vi "Bertta_v09_97.vi"() -> ()   [LabVIEW 2016]
uses:
  x64/Debug/BERTTA.dll
panel:
  out "element":bool
  out "Started:":string
  in  "SHUTDOWN":bool
  in  "MASTER CONTROL":bool
  in  "Tab Control":T1(tab)
  out "Output File":path caption="selected path"
  in  "Browse folder":path=path "" caption="start path"
  in  "Read Seq":bool
  in  "Save Seq":bool
  in  "Configuration file":path=path "C:/Users/shresplab/Desktop/BerttaConfiguration.lvm" caption="Filename"
  in  "OK Button 2":bool
  out "Boolean":bool
  in  "User (initials)":string
  in  "Project name":string
  in  "Description":string
  out "PUMP1":bool
  out "Target amount":dbl
  out "Scale weight":dbl
  out "Amount now":dbl
  out "Flow rate":dbl
  out "Time to target":dbl format="%<%H:%M:%S>t"
  out "Current step":dbl
  out "Target":dbl
  out "Amount now":dbl
  out "Amount now":dbl
  out "Target":dbl
  out "Current step":dbl
  out "Time to target":dbl format="%<%H:%M:%S>t"
  out "Flow rate":dbl
  out "Amount now":dbl
  out "Scale weight":dbl
  out "Target amount":dbl
  out "PUMP2":bool
  out "Sensor OK 6":bool
  out "Sensor OK 5":bool
  out "Sensor OK 4":bool
  out "Sensor OK 3":bool
  in  "OK Button":bool
  in  "Add comment":string
  out "PUMP3":bool
  out "Target amount":dbl
  out "Scale weight":dbl
  out "Amount now":dbl
  out "Flow rate":dbl
  out "Time to target":dbl format="%<%H:%M:%S>t"
  out "Current step":dbl
  out "Target":dbl
  out "Amount now":dbl
  out "Tr":dbl
  out "Tj in":dbl
  out "Tj out":dbl
  out "T set":dbl
  out "Current step":i32
  out "RPM":dbl
  out "Torque 2":dbl
  out "Waveform Chart 5":dynamicdata(graph)
  out "Waveform Chart 6":dynamicdata(graph)
  out "Waveform Chart 7":dynamicdata(graph)
  in  "Tab Control 2":T2(tab)
  out "Waveform Chart 3":dynamicdata(graph)
  out "Waveform Chart 8":dynamicdata(graph)
  out "Waveform Chart 11":dynamicdata(graph)
  out "Waveform Chart 13":dynamicdata(graph)
  out "Waveform Chart 9":dynamicdata(graph)
  out "Table":string[][](table)=[["14.8.2017 18.06.59", "0,000000", "417,670000", "-0,150000", "1,000000", "22,220000", "23,366837", "23,574959", "23,985852", "23,690000", "240,000000", "4,000000", "0,000000", "397,000000", "-397,000000", "1,000000"], ["14.8.2017 18.07.06", "0,000000", "417,640000", "-0,120000", "1,000000", "22,220000", "23,763115", "23,906257", "23,985694", "23,680000", "240,000000", "4,000000", "0,000000", "397,000000", "-397,000000", "1,000000"], ["14.8.2017 18.07.13", "0,000000", "417,640000", "-0,120000", "1,000000", "22,220000", "23,965922", "24,013440", "23,984906", "23,670000", "240,000000", "4,100000", "3,000000", "397,000000", "-397,000000", "1,000000"], ["14.8.2017 18.07.21", "0,000000", "417,640000", "-0,120000", "1,000000", "22,220000", "23,943860", "23,900110", "23,987113", "23,670000", "240,000000", "4,000000", "0,000000", "397,000000", "-397,000000", "1,000000"], ["14.8.2017 18.07.28", "0,000000", "417,640000", "-0,120000", "1,000000", "22,220000", "23,736328", "23,600018", "23,989004", "23,660000", "240,000000", "4,000000", "0,000000", "397,000000", "-397,000000", "1,000000"], ["14.8.2017 18.07.36", "0,000000", "417,640000", "-0,120000", "1,000000", "22,220000", "23,480910", "23,324538", "23,991053", "23,660000", "240,000000", "4,000000", "0,000000", "397,000000", "-397,000000", "1,000000"], ["14.8.2017 18.07.43", "0,000000", "417,640000", "-0,120000", "2,000000", "22,220000", "23,195579", "23,008270", "23,999093", "23,650000", "240,000000", "4,000000", "0,000000", "397,000000", "-397,000000", "1,000000"], ["14.8.2017 18.07.51", "0,000000", "417,650000", "-417,650000", "1,000000", "22,220000", "22,862541", "22,649021", "24,003979", "23,650000", "240,000000", "4,000000", "0,000000", "397,000000", "-397,000000", "2,000000"], ["14.8.2017 18.07.58", "0,000000", "417,640000", "0,010000", "1,000000", "22,220000", "22,541353", "22,354878", "24,005398", "23,650000", "240,000000", "4,000000", "0,000000", "397,000000", "-397,000000", "1,000000"], ["14.8.2017 18.08.06", "0,000000", "417,640000", "0,010000", "1,000000", "22,220000", "22,347931", "22,253738", "24,007605", "23,640000", "240,000000", "4,100000", "0,000000", "397,000000", "-397,000000", "1,000000"], ["14.8.2017 18.08.13", "0,000000", "417,640000", "0,010000", "1,000000", "22,220000", "22,329030", "22,302102", "24,006028", "23,640000", "240,000000", "4,000000", "0,000000", "395,820000", "-395,820000", "1,000000"], ["14.8.2017 18.08.20", "0,000000", "417,640000", "0,010000", "1,000000", "22,220000", "22,466849", "22,511320", "24,002403", "23,630000", "240,000000", "4,000000", "0,000000", "395,830000", "-0,010000", "1,000000"], ["14.8.2017 18.08.28", "0,000000", "417,640000", "0,010000", "1,000000", "22,220000", "22,707062", "22,835101", "24,000984", "23,620000", "240,000000", "4,000000", "0,000000", "395,830000", "-0,010000", "1,000000"], ["14.8.2017 18.08.35", "0,000000", "417,640000", "0,010000", "1,000000", "22,220000", "23,054104", "23,232979", "24,001299", "23,600000", "240,000000", "4,000000", "0,000000", "395,830000", "-0,010000", "1,000000"], ["14.8.2017 18.08.43", "0,000000", "417,640000", "0,010000", "1,000000", "22,220000", "23,412371", "23,522793", "24,002560", "23,590000", "240,000000", "4,000000", "0,000000", "395,820000", "0,000000", "1,000000"], ["14.8.2017 18.08.51", "0,000000", "417,640000", "0,010000", "1,000000", "22,220000", "23,596247", "23,656125", "24,003821", "23,580000", "240,000000", "4,000000", "0,000000", "395,820000", "0,000000", "1,000000"]]
  out "Boolean 4":bool
  out "Boolean 3":bool
  out "Boolean 2":bool
  in  "Reset 6":bool
  in  "Manual/Ramp":bool=TRUE
  in  "Array":dbl[][](array[numeric])=[[20.0, 0.0], [20.0, 0.0], [20.0, 0.0]]
  in  "?":bool
  in  "Time":dbl format="Time to target (min):                %#_g"
  out "Current temp":dbl format="Current temperature (S1):   %#_6g"
  in  "OK Button 3":bool
  in  "T ext / T ext 2":enum32{"Sensor 1", "Sensor 2"}(radio)
  out "Sensor OK":bool
  in  "T fail":dbl=20.0 format="Failsafe temperature:              %#_g"
  in  "Setpoint":dbl=20.0 format="Temperature target:                %#_6g"
  in  "Manual select":T3(radio)
  out "Waveform Chart":dynamicdata(graph)
  out "T external 2":dbl format="Current temperature (S2):    %#_g"
  in  "UPDATE TEMP":bool
  out "Led11 5":bool
  out "RPM":dbl format="%_4f"
  out "Led10 3":bool
  out "Led9 3":bool
  out "Led8 3":bool
  out "Led7 3":bool
  out "Led6 3":bool
  out "Led5 3":bool
  out "Led4 3":bool
  out "Led3 3":bool
  out "Led2 3":bool
  out "Led1 3":bool
  in  "PumpSeq 4":dbl[][](array[numeric])=[[0.0, 0.0, 0.0, 0.0, 0.0, 0.0, 0.0, 0.0, 0.0, 0.0], [0.0, 0.0, 0.0, 0.0, 0.0, 0.0, 0.0, 0.0, 0.0, 0.0], [0.0, 0.0, 0.0, 0.0, 0.0, 0.0, 0.0, 0.0, 0.0, 0.0], [0.0, 0.0, 0.0, 0.0, 0.0, 0.0, 0.0, 0.0, 0.0, 0.0], [0.0, 0.0, 0.0, 0.0, 0.0, 0.0, 0.0, 0.0, 0.0, 0.0], [0.0, 0.0, 0.0, 0.0, 0.0, 0.0, 0.0, 0.0, 0.0, 0.0], [0.0, 0.0, 0.0, 0.0, 0.0, 0.0, 0.0, 0.0, 0.0, 0.0], [0.0, 0.0, 0.0, 0.0, 0.0, 0.0, 0.0, 0.0, 0.0, 0.0], [0.0, 0.0, 0.0, 0.0, 0.0, 0.0, 0.0, 0.0, 0.0, 0.0], [0.0, 0.0, 0.0, 0.0, 0.0, 0.0, 0.0, 0.0, 0.0, 0.0]]
  in  "?":bool
  out "Flow rate (g/min)":dbl
  out "Scale reading":dbl
  out "Step amount now":dbl
  in  "Grams / min":dbl
  out "Waveform Chart 14":dynamicdata(graph)
  in  "?":bool
  out "Total amount now":dbl
  out "Led11 4":bool
  in  "Reset 5":bool
  out "Elapsed / step":i32
  out "Time to target":dbl format="%<%H:%M:%S>t"
  in  "OK Button 4":bool
  out "Led11":bool
  out "RPM":dbl format="%_4f"
  out "Led10":bool
  out "Led9":bool
  out "Led8":bool
  out "Led7":bool
  out "Led6":bool
  out "Led5":bool
  out "Led4":bool
  out "Led3":bool
  out "Led2":bool
  out "Led1":bool
  in  "PumpSeq 2":dbl[][](array[numeric])=[[0.0, 0.0, 0.0, 0.0, 0.0, 0.0, 0.0, 0.0, 0.0, 0.0], [0.0, 0.0, 0.0, 0.0, 0.0, 0.0, 0.0, 0.0, 0.0, 0.0], [0.0, 0.0, 0.0, 0.0, 0.0, 0.0, 0.0, 0.0, 0.0, 0.0], [0.0, 0.0, 0.0, 0.0, 0.0, 0.0, 0.0, 0.0, 0.0, 0.0], [0.0, 0.0, 0.0, 0.0, 0.0, 0.0, 0.0, 0.0, 0.0, 0.0], [0.0, 0.0, 0.0, 0.0, 0.0, 0.0, 0.0, 0.0, 0.0, 0.0], [0.0, 0.0, 0.0, 0.0, 0.0, 0.0, 0.0, 0.0, 0.0, 0.0], [0.0, 0.0, 0.0, 0.0, 0.0, 0.0, 0.0, 0.0, 0.0, 0.0], [0.0, 0.0, 0.0, 0.0, 0.0, 0.0, 0.0, 0.0, 0.0, 0.0], [0.0, 0.0, 0.0, 0.0, 0.0, 0.0, 0.0, 0.0, 0.0, 0.0]]
  in  "?":bool
  out "Flow rate (g/min)":dbl
  out "Scale reading":dbl
  out "Step amount now":dbl
  in  "Grams / min":dbl
  out "Waveform Chart 10":dynamicdata(graph)
  in  "?":bool
  out "Total amount now":dbl
  out "Led11":bool
  in  "Reset 3":bool
  out "Elapsed / step":i32
  out "Time to target":dbl format="%<%H:%M:%S>t"
  in  "OK Button 5":bool
  out "Led11 3":bool
  out "RPM":dbl format="%_4f"
  out "Led10 2":bool
  out "Led9 2":bool
  out "Led8 2":bool
  out "Led7 2":bool
  out "Led6 2":bool
  out "Led5 2":bool
  out "Led4 2":bool
  out "Led3 2":bool
  out "Led2 2":bool
  out "Led1 2":bool
  in  "PumpSeq 3":dbl[][](array[numeric])=[[0.0, 0.0, 0.0, 0.0, 0.0, 0.0, 0.0, 0.0, 0.0, 0.0], [0.0, 0.0, 0.0, 0.0, 0.0, 0.0, 0.0, 0.0, 0.0, 0.0], [0.0, 0.0, 0.0, 0.0, 0.0, 0.0, 0.0, 0.0, 0.0, 0.0], [0.0, 0.0, 0.0, 0.0, 0.0, 0.0, 0.0, 0.0, 0.0, 0.0], [0.0, 0.0, 0.0, 0.0, 0.0, 0.0, 0.0, 0.0, 0.0, 0.0], [0.0, 0.0, 0.0, 0.0, 0.0, 0.0, 0.0, 0.0, 0.0, 0.0], [0.0, 0.0, 0.0, 0.0, 0.0, 0.0, 0.0, 0.0, 0.0, 0.0], [0.0, 0.0, 0.0, 0.0, 0.0, 0.0, 0.0, 0.0, 0.0, 0.0], [0.0, 0.0, 0.0, 0.0, 0.0, 0.0, 0.0, 0.0, 0.0, 0.0], [0.0, 0.0, 0.0, 0.0, 0.0, 0.0, 0.0, 0.0, 0.0, 0.0]]
  in  "?":bool
  out "Flow rate (g/min)":dbl
  out "Scale reading":dbl
  out "Step amount now":dbl
  in  "Grams / min":dbl
  out "Waveform Chart 12":dynamicdata(graph)
  in  "?":bool
  out "Total amount now":dbl
  out "Led11 2":bool
  in  "Reset 4":bool
  out "Elapsed / step":i32
  out "Time to target":dbl format="%<%H:%M:%S>t"
  in  "OK Button 6":bool
  in  "Remote / Manual":bool
  in  "Set RPM":i32
  out "RPM":dbl
  out "Torque":dbl
  out "Waveform Chart 4":dynamicdata(graph)
  in  "OK Button 7":bool
  out "PortDev out":dbl[](array[numeric])
  in  "Save PortDev":bool
  out "PortDev in":dbl[](array[numeric])
  in  "dev1":i32
  in  "dev2":i32
  in  "dev3":i32
  in  "dev4":i32
  in  "dev5":i32
  in  "dev6":i32
  in  "dev8":i32
  in  "port1":i32
  in  "port2":i32
  in  "port3":i32
  in  "port4":i32
  in  "port5":i32
  in  "port6":i32
  in  "port7":i32
  in  "port8":i32
  in  "dev7":i32
  in  "Treshold (T/C)":dbl=0.5
  out "DAQ 9217 (PT100)":errorcluster
  out "Config File":dbl[][](array[numeric])
  # "Temperature sensor:"
  # "Manual control:"
  # "PUMP & SCALE 1"
  # "STEP"
  # "TOTAL"
  # "PUMP & SCALE 2"
  # "STEP"
  # "TOTAL"
  # "PUMP & SCALE 3"
  # "STEP"
  # "TOTAL"
  # "Temperature control parameter"
  # "Secondary temperature sensor"
  # "Temp target"
  # "Time target"
  # "Grams    /   min"
  # "End of sequence"
  # "Manual control"
  # "Grams    /   min"
  # "End of sequence"
  # "Manual control"
  # "Grams    /   min"
  # "End of sequence"
  # "Manual control"
  # "dev1 and dev2 always to port1 and 2\nport1 = port2 = Lauda\n\ndev3 and dev4 always to port3 and port4\nport3 = port4 = Heidolph"
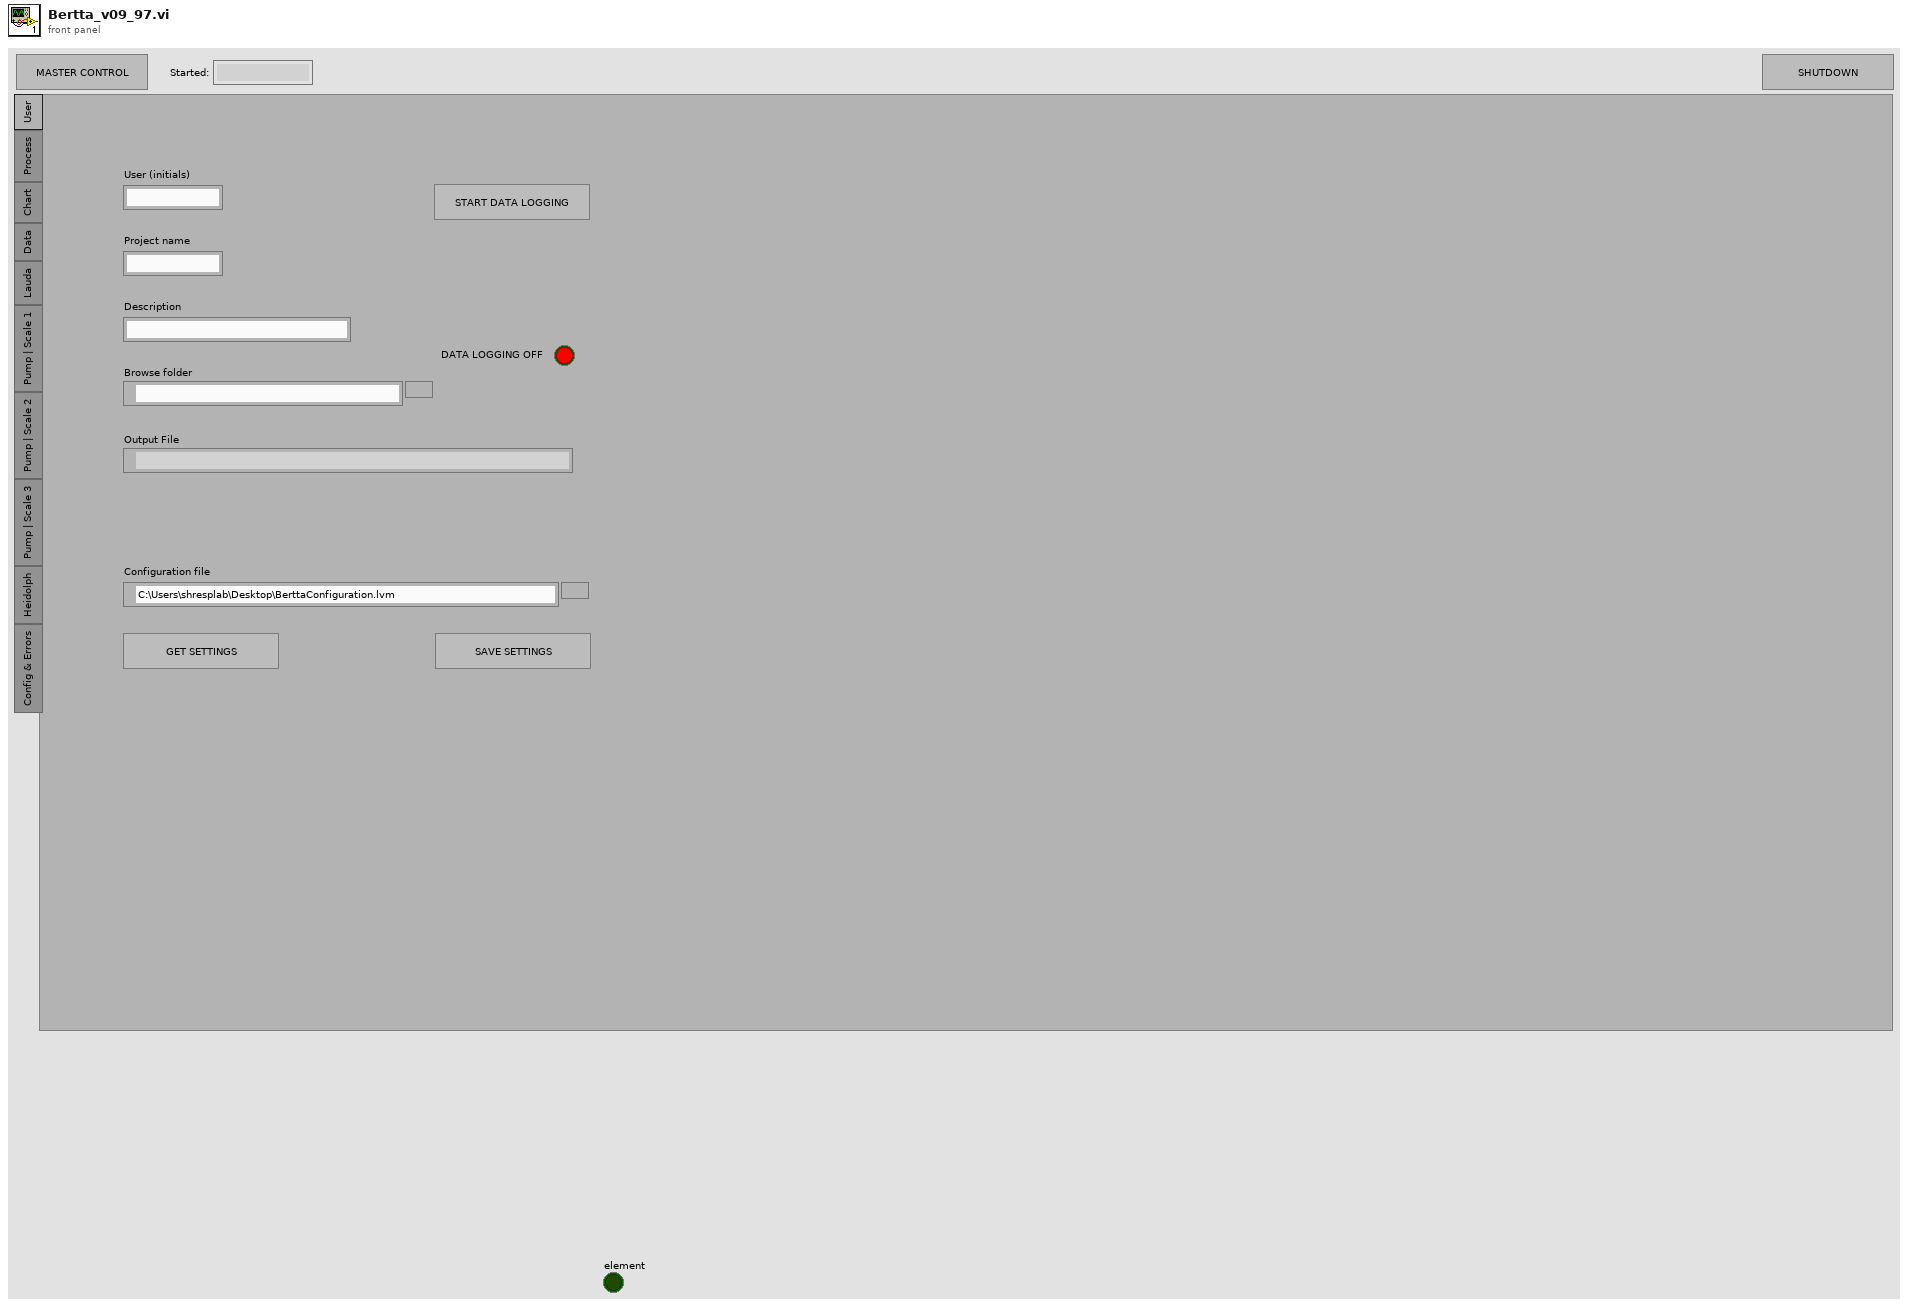
[diagram p1: front panel]
types:
  T1 = enum32{"User", "Process", "Chart", "Data", "Lauda", "Pump | Scale 1", "Pump | Scale 2", "Pump | Scale 3", "Heidolph", "Config & Errors"}
  T2 = enum32{"Temperatures", "Scale / Pump 1", "Scale / Pump 2", "Scale / Pump 3", "RPM / torque"}
  T3 = enum32{"Reactor temperature", "Jacket temperature"}
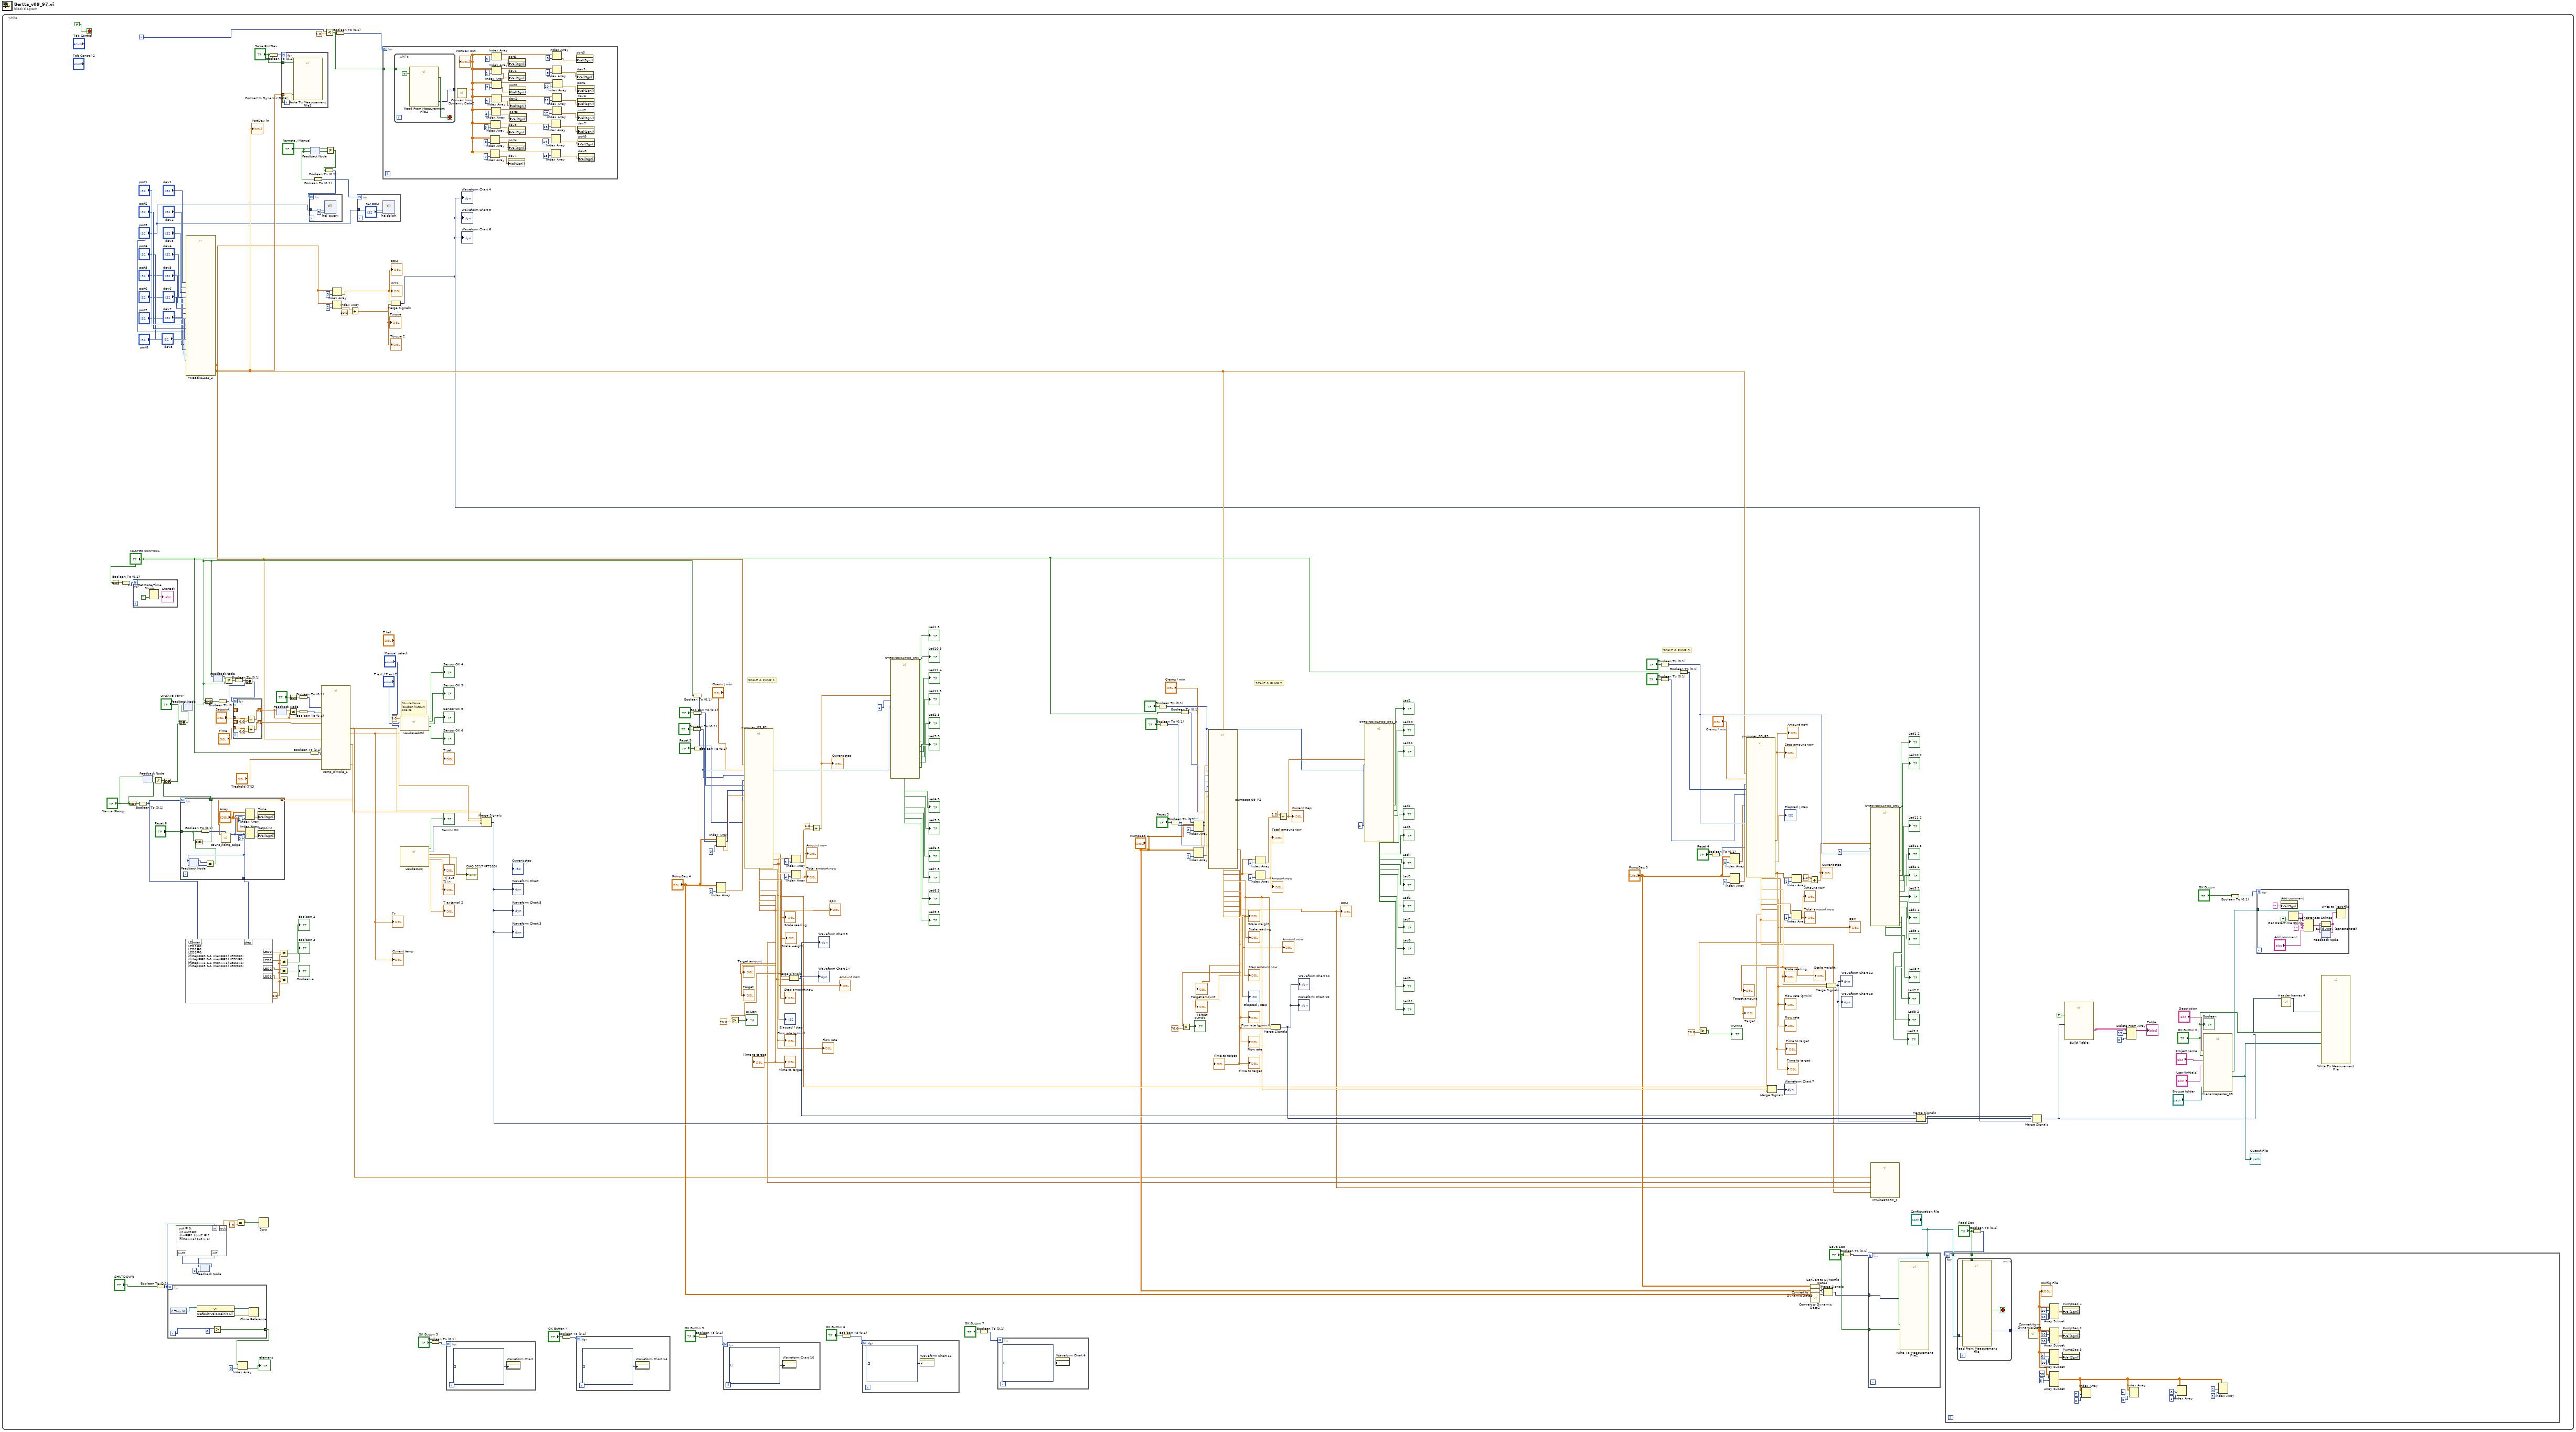
[diagram p0: block diagram]
diagram:
  n1 = while {
    i -> [w42]
    stop <- FALSE stop-if-true
    w28 = 0.0 ("y")
    # "Muutettava\nlaudan kutsun \nosalta"
    # "SCALE & PUMP 1"
    # "SCALE & PUMP 3"
    # "SCALE & PUMP 2"
    n2 = Not(x="MASTER CONTROL") -> (.not. x?=w274:bool)
    n3 = Boolean To (0,1)(Boolean=w274) -> (0, 1=w275:i16)
    n4 = Not(x="Manual/Ramp") -> (.not. x?=w35:bool)
    n5 = for {
      N: w275 -> [_]
      n6 = Get Date/Time String(want seconds? (F)=TRUE) -> (time string=→"Started:":string)  [unwired: 2 in, 1 out]
    }
    n7 = Boolean To (0,1)(Boolean=w35) -> (0, 1=w17:i16)
    n8 = feedback #1() -> (w23:bool)  [unwired: 1 in]
    n9 = feedback-in #1("Manual/Ramp") -> ()
    n10 = Not Equal?(x=w23, y="Manual/Ramp") -> (x != y?=w20:bool)
    n11 = Boolean To (0,1)(Boolean="SHUTDOWN") -> (0, 1=w259:i16)
    n12 = for {
      N: w259 -> [_]
      tunnel: [w390] -> w273 mode=indexing
      i -> [w392]
      n13 = control-ref of="This VI"() -> (w395:refnum<vi>)
      n14 = invoke class="VI" method="Default Vals.Reinit All"(reference=w395) -> (reference out=w393:refnum<vi>, error out=w394:errorcluster)  [unwired: 2 in, 1 out]
      n15 = Greater?(x=w392, y=0) -> (0:w390:bool)
      n16 = Close Reference(reference=w393, error in (no error)=w394) -> ()  [unwired: 1 out]
    }
    n17 = feedback #2() -> (w15:bool)  [unwired: 1 in]
    n18 = call "MReadRS232_2.vi"("port1"="port1", "dev1"="dev1", "port2"="port2", "dev2"="dev2", "port3"="port3", "dev7"="dev7", "dev8"="dev8", "port7"="port7", "port8"="port8", "dev5"="dev5", "port5"="port5", "dev4"="dev4", "dev6"="dev6", "port6"="port6", "port4"="port4", "dev3"="dev3") -> ("output array"=w46:dbl[], "params"=w7:dbl[])  [unwired: 2 in]
    "PortDev in" <- w46
    n19 = feedback #3(0) -> (w257:i32)
    n20 = formula code="out = 0;\nint out2=0;\nif(in==1 ) out2 = 1;\nif(in2==1) out = 1;"("in"=w259, "in2"=w257) -> ("out"=w261:dbl, "out2"=w258:i32)
    n21 = feedback-in #3(w258) -> ()
    n22 = And(x="MASTER CONTROL", y=w15) -> (x .and. y?=w75:bool)
    n23 = feedback #4() -> (w66:bool)  [unwired: 1 in]
    n24 = feedback-in #4("MASTER CONTROL") -> ()
    n25 = Boolean To (0,1)(Boolean=w75) -> (0, 1=w63:i16)
    n26 = Not Equal?(x=w66, y="MASTER CONTROL") -> (x != y?=w65:bool)
    n27 = Boolean To (0,1)(Boolean=w65) -> (0, 1=w62:i16)
    n28 = Equal?(x=w261, y=1.0) -> (x = y?=w260:bool)
    n29 = Index Array(array=w273, index=0) -> (element=→"element":bool)
    n30 = Or(x=w62, y=w63) -> (x .or. y?=w61:i16)
    n31 = for {
      N: w61 -> [_]
      tunnel: "Time" -> [w342]
      shift-right: [w341] -> w76
      shift-left: _ -> [_]
      tunnel: "Setpoint" -> [w339]
      shift-right: [w338] -> w73
      shift-left: _ -> [_]
      n32 = Add(x=w339, y=0.0) -> (x+y=w338:dbl)
      n33 = Add(x=w342, y=0.0) -> (x+y=w341:dbl)
    }
    n34 = Stop(stop? (T)=w260) -> ()
    n35 = Boolean To (0,1)(Boolean="Save PortDev") -> (0, 1=w45:i16)
    n36 = feedback-in #5(w73) -> ()
    n37 = feedback #5() -> (w74:dbl)  [unwired: 1 in]
    n38 = for {
      N: w45 -> [_]
      tunnel: w46 -> [w337]
      tunnel: "Save PortDev" -> [w335]
      n39 = call "Convert to Dynamic Data"("Array"=w337) -> ("Dynamic Data Type"=w336:dynamicdata)  [unwired: 3 in]
      n40 = call "Write To Measurement File3"("Signals"=w336, "Reset"=w335) -> ()  [unwired: 15 in, 3 out]
    }
    n41 = Not(x="?") -> (.not. x?=w69:bool)
    n42 = Not Equal?(x=w74, y=w73) -> (x != y?=w72:bool)
    n43 = Boolean To (0,1)(Boolean=w69) -> (0, 1=w71:i16)
    n44 = Boolean To (0,1)(Boolean=w72) -> (0, 1=w67:i16)
    n45 = Boolean To (0,1)(Boolean="MASTER CONTROL") -> (0, 1=w68:i16)
    n46 = feedback-in #6("Remote / Manual") -> ()
    n47 = feedback #6() -> (w12:bool)  [unwired: 1 in]
    n48 = Boolean To (0,1)(Boolean="Remote / Manual") -> (0, 1=w10:i16)
    n49 = call "ramp_simple_1.vi"("array"=w7, "treshold"="Treshold (T/C)", "time_set"=w76, "T_sp"=w73, "master"=w68, "reset"=w67, "pause"=w71) -> ("T control"=w81:dbl, "Tr"=w80:dbl, "Tin"=w79:dbl, "target_reached"=w33:dbl)  [unwired: 1 out]
    "Tr" <- w80
    "Current temp" <- w80
    n50 = for {
      N: w17 -> [_]
      tunnel: w33 -> [w294]
      tunnel: [w284] -> w21
      tunnel: "Reset 6" -> [w286]
      tunnel: [w287] -> w24
      n51 = feedback #7() -> (w288:i32)  [unwired: 1 in]
      n52 = Boolean To (0,1)(Boolean=w286) -> (0, 1=w289:i16)
      n53 = call "count_rising_edge.vi"("reset"=w289, "target_reached"=w294) -> ("element 2"=w287:i32)  [unwired: 9 in]
      n54 = feedback-in #7(w287) -> ()
      n55 = Not Equal?(x=w288, y=w287) -> (x != y?=w285:bool)
      n56 = Or(x=w286, y=w285) -> (x .or. y?=w284:bool)
      n57 = Index Array(array="Array", index (row)=w287, index (col)=1 ("disabled index (col)")) -> (element=w290:dbl)
      n58 = Index Array(array="Array", index (row)=w287, index (col)=0 ("disabled index (col)")) -> (element=w291:dbl)
      n59 = property on="Time" class="DigNum (strict)"("Val(Sgnl)"=w290) -> ()  [unwired: 2 in, 2 out]
      n60 = property on="Setpoint" class="DigNum (strict)"("Val(Sgnl)"=w291) -> ()  [unwired: 2 in, 2 out]
    }
    n61 = Or(x=w20, y=w21) -> (x .or. y?=w19:bool)
    n62 = Or(x="UPDATE TEMP", y=w19) -> (x .or. y?=w16:bool)
    n63 = feedback-in #2(w16) -> ()
    n64 = formula code="LED0=0;\nLED1=0;\nLED2=0;\nLED3=0;\nif(step==0 && man==1) LED0=1;\nif(step==1 && man==1) LED1=1;\nif(step==2 && man==1) LED2=1;\nif(step==3 && man==1) LED3=1;"("step"=w24, "man"=w17) -> ("LED0"=w32:dbl, "LED1"=w31:dbl, "LED2"=w30:dbl, "LED3"=w29:dbl)
    n65 = Not Equal?(x=w32, y=w28) -> (x != y?=→"Boolean 2":bool)
    n66 = Not Equal?(x=w31, y=w28) -> (x != y?=→"Boolean 3":bool)
    n67 = Not Equal?(x=w30, y=w28) -> (x != y?=→"Boolean 4":bool)
    n68 = Not Equal?(x=w29, y=w28) -> ()  [unwired: 1 out]
    n69 = Less?(x=w42, y=1.0) -> (x < y?=w40:bool)
    n70 = Not Equal?(x=w12, y="Remote / Manual") -> (x != y?=w11:bool)
    n71 = Boolean To (0,1)(Boolean=w11) -> (0, 1=w13:i16)
    n72 = for {
      N: w13 -> [_]
      tunnel: "port3" -> [w282]
      n73 = dll-call lib="C:/Users/shresplab/OneDrive - Kemira Oyj/Documents/GitHub/Bertta/BERTTA/x64/Debug/BERTTA.dll" fn="hei_query"("port"=w282, "q"=5) -> ()  [unwired: 6 in, 2 out]
    }
    n74 = Index Array(array=w7, index=3) -> (element=w4:dbl)
    "RPM" <- w4
    "RPM" <- w4
    n75 = Index Array(array=w7, index=2) -> (element=w6:dbl)
    n76 = Boolean To (0,1)(Boolean=w40) -> (0, 1=w41:i16)
    n77 = Divide(x=w6, y=10.0) -> (x/y=w3:dbl)
    "Torque" <- w3
    "Torque 2" <- w3
    n78 = for {
      N: w10 -> [_]
      tunnel: "port3" -> [w280]
      n79 = dll-call lib="C:/Users/shresplab/OneDrive - Kemira Oyj/Documents/GitHub/Bertta/BERTTA/x64/Debug/BERTTA.dll" fn="heidolph"("port"=w280, "speed"="Set RPM") -> ()  [unwired: 6 in, 2 out]
    }
    n80 = for {
      N: w41 -> [_]
      tunnel: w40 -> [w330]
      n81 = while {
        tunnel: [w333] -> w329
        tunnel: w330 -> [w331]
        stop <- w334 stop-if-true
        n82 = call "Read From Measurement File2"("Enable"=TRUE, "Reset"=w331) -> ("Signals"=w333:dynamicdata, "EOF?"=w334:bool)  [unwired: 4 in, 4 out]
      }
      n83 = call "Convert from Dynamic Data2"("Dynamic Data Type"=w329) -> ("Array"=w312:dbl[])  [unwired: 3 in]
      "PortDev out" <- w312
      n84 = Index Array(array=w312, index=6) -> (element=w305:dbl)
      n85 = Index Array(array=w312, index=7) -> (element=w304:dbl)
      n86 = Index Array(array=w312, index=5) -> (element=w306:dbl)
      n87 = Index Array(array=w312, index=4) -> (element=w307:dbl)
      n88 = Index Array(array=w312, index=0) -> (element=w311:dbl)
      n89 = Index Array(array=w312, index=1) -> (element=w310:dbl)
      n90 = Index Array(array=w312, index=3) -> (element=w308:dbl)
      n91 = Index Array(array=w312, index=2) -> (element=w309:dbl)
      n92 = property on="dev4" class="DigNum (strict)"("Val(Sgnl)"=w304) -> ()  [unwired: 2 in, 2 out]
      n93 = property on="dev3" class="DigNum (strict)"("Val(Sgnl)"=w306) -> ()  [unwired: 2 in, 2 out]
      n94 = property on="port4" class="DigNum (strict)"("Val(Sgnl)"=w305) -> ()  [unwired: 2 in, 2 out]
      n95 = property on="port1" class="DigNum (strict)"("Val(Sgnl)"=w311) -> ()  [unwired: 2 in, 2 out]
      n96 = property on="dev1" class="DigNum (strict)"("Val(Sgnl)"=w310) -> ()  [unwired: 2 in, 2 out]
      n97 = property on="port2" class="DigNum (strict)"("Val(Sgnl)"=w309) -> ()  [unwired: 2 in, 2 out]
      n98 = property on="dev2" class="DigNum (strict)"("Val(Sgnl)"=w308) -> ()  [unwired: 2 in, 2 out]
      n99 = property on="port3" class="DigNum (strict)"("Val(Sgnl)"=w307) -> ()  [unwired: 2 in, 2 out]
      n100 = Index Array(array=w312, index=14) -> (element=w297:dbl)
      n101 = Index Array(array=w312, index=15) -> (element=w296:dbl)
      n102 = Index Array(array=w312, index=13) -> (element=w298:dbl)
      n103 = Index Array(array=w312, index=12) -> (element=w299:dbl)
      n104 = Index Array(array=w312, index=8) -> (element=w303:dbl)
      n105 = Index Array(array=w312, index=9) -> (element=w302:dbl)
      n106 = Index Array(array=w312, index=11) -> (element=w300:dbl)
      n107 = Index Array(array=w312, index=10) -> (element=w301:dbl)
      n108 = property on="port5" class="DigNum (strict)"("Val(Sgnl)"=w303) -> ()  [unwired: 2 in, 2 out]
      n109 = property on="dev5" class="DigNum (strict)"("Val(Sgnl)"=w302) -> ()  [unwired: 2 in, 2 out]
      n110 = property on="port6" class="DigNum (strict)"("Val(Sgnl)"=w301) -> ()  [unwired: 2 in, 2 out]
      n111 = property on="dev6" class="DigNum (strict)"("Val(Sgnl)"=w300) -> ()  [unwired: 2 in, 2 out]
      n112 = property on="port7" class="DigNum (strict)"("Val(Sgnl)"=w299) -> ()  [unwired: 2 in, 2 out]
      n113 = property on="dev7" class="DigNum (strict)"("Val(Sgnl)"=w298) -> ()  [unwired: 2 in, 2 out]
      n114 = property on="port8" class="DigNum (strict)"("Val(Sgnl)"=w297) -> ()  [unwired: 2 in, 2 out]
      n115 = property on="dev8" class="DigNum (strict)"("Val(Sgnl)"=w296) -> ()  [unwired: 2 in, 2 out]
    }
    n116 = Merge Signals(w4, w3) -> (w2:dynamicdata)
    "Waveform Chart 4" <- w2
    "Waveform Chart 6" <- w2
    "Waveform Chart 9" <- w2
    n117 = call "LaudaLedCtrl.vi"("Manual select"="Manual select", "T ext / T ext in"="T ext / T ext 2", "Lauda port"=9.0) -> ("Sensor OK 5"=→"Sensor OK 5":bool, "Sensor OK 3"=→"Sensor OK 3":bool, "Sensor OK 4"=→"Sensor OK 4":bool, "Sensor OK 6"=→"Sensor OK 6":bool)  [unwired: 5 in]
    n118 = call "LaudaDAQ.vi"() -> ("error out"=→"DAQ 9217 (PT100)":errorcluster, 1:"Tj out"=→"Tj out":dbl, "data"=w149:dynamicdata, "Sensor OK"=→"Sensor OK":bool, 4:"Tj out"=→"Tj in":dbl, "T external 2"=→"T external 2":dbl)  [unwired: 6 in]
    n119 = Boolean To (0,1)(Boolean="OK Button 3") -> (0, 1=w92:i16)
    n120 = for {
      N: w92 -> [_]
      n121 = property on="Waveform Chart" class="WFChart (strict)"("History Data"=dynamicdata[] []) -> ()  [unwired: 2 in, 2 out]
    }
    n122 = Merge Signals(w81, w80, w79, w149) -> (w150:dynamicdata)
    "Waveform Chart 3" <- w150
    "Waveform Chart" <- w150
    "Waveform Chart 5" <- w150
    n123 = Boolean To (0,1)(Boolean="OK Button 4") -> (0, 1=w90:i16)
    n124 = for {
      N: w90 -> [_]
      n125 = property on="Waveform Chart 14" class="WFChart (strict)"("History Data"=dynamicdata[] []) -> ()  [unwired: 2 in, 2 out]
    }
    n126 = Boolean To (0,1)(Boolean="?") -> (0, 1=w158:i16)
    n127 = Boolean To (0,1)(Boolean="?") -> (0, 1=w162:i16)
    n128 = Boolean To (0,1)(Boolean="MASTER CONTROL") -> (0, 1=w154:i16)
    n129 = Boolean To (0,1)(Boolean="Reset 5") -> (0, 1=w161:i16)
    n130 = Boolean To (0,1)(Boolean="OK Button 5") -> (0, 1=w88:i16)
    n131 = Index Array(array="PumpSeq 4", index (col)=0) -> (element=w166:dbl[])  [unwired: 1 in]
    n132 = Index Array(array="PumpSeq 4", index (col)=1) -> (element=w187:dbl[])  [unwired: 1 in]
    n133 = for {
      N: w88 -> [_]
      n134 = property on="Waveform Chart 10" class="WFChart (strict)"("History Data"=dynamicdata[] []) -> ()  [unwired: 2 in, 2 out]
    }
    n135 = call "pumpsec_09_P1.vi"("reset"=w161, "master"=w154, "manual"=w158, "pause"=w162, "Array"=w7, "Target"=w166, "fr_manual"="Grams / min", "Time"=w187) -> ("pumpCtrl"=w133:dbl, "totaltarget"=→"Target":dbl, "target_step"=→"Target amount":dbl, "REGLO D"=w99:dbl, "time_to_target"=→"Time to target" →"Time to target":dbl, "step_fr"=w110:dbl, "amount_step"=→"Amount now" →"Step amount now":dbl, "Scale"=w145:dbl, "elapsed_step"=→"Elapsed / step":dbl, "params"=w184:dbl[])  [unwired: 8 in, 2 out]
    "Flow rate" <- w110
    "Scale weight" <- w145
    "Scale reading" <- w145
    "Flow rate (g/min)" <- w110
    "RPM" <- w99
    n136 = Greater?(x=w133, y=70.0) -> (0:→"PUMP1":bool)
    n137 = Merge Signals(w145, w110) -> (w153:dynamicdata)
    "Waveform Chart 8" <- w153
    "Waveform Chart 14" <- w153
    n138 = Index Array(array=w184, index=1) -> (element=w181:dbl)
    n139 = Index Array(array=w184, index=2) -> (element=→"Amount now" →"Total amount now":dbl)
    n140 = Add(x=1.0, y=w181) -> (x+y=w111:dbl)
    "Current step" <- w111
    n141 = Boolean To (0,1)(Boolean="OK Button 6") -> (0, 1=w86:i16)
    n142 = for {
      N: w86 -> [_]
      n143 = property on="Waveform Chart 12" class="WFChart (strict)"("History Data"=dynamicdata[] []) -> ()  [unwired: 2 in, 2 out]
    }
    n144 = call "STEPINDICATOR_091_2.vi"("current step"=w111, "enable"=i16 1, "manual"=w158) -> ("Led 8"=→"Led8 3":bool, "Led 10"=→"Led10 3":bool, "Led 11"=→"Led11 4":bool, "Led 7"=→"Led7 3":bool, "Led 1"=→"Led1 3":bool, "Led 6"=→"Led6 3":bool, "Led 2"=→"Led2 3":bool, "Led 12"=→"Led11 5":bool, "Led 5"=→"Led5 3":bool, "Led 4"=→"Led4 3":bool, "Led 3"=→"Led3 3":bool, "Led 9"=→"Led9 3":bool)  [unwired: 1 in]
    n145 = Boolean To (0,1)(Boolean="OK Button 7") -> (0, 1=w84:i16)
    n146 = for {
      N: w84 -> [_]
      n147 = property on="Waveform Chart 4" class="WFChart (strict)"("History Data"=dynamicdata[] []) -> ()  [unwired: 2 in, 2 out]
    }
    n148 = Boolean To (0,1)(Boolean="?") -> (0, 1=w221:i16)
    n149 = Boolean To (0,1)(Boolean="?") -> (0, 1=w248:i16)
    n150 = Boolean To (0,1)(Boolean="Reset 3") -> (0, 1=w246:i16)
    n151 = Boolean To (0,1)(Boolean="MASTER CONTROL") -> (0, 1=w240:i16)
    n152 = Index Array(array="PumpSeq 2", index (col)=0 ("disabled index (col)")) -> (element=w251:dbl[])  [unwired: 1 in]
    n153 = Index Array(array="PumpSeq 2", index (col)=1 ("disabled index (col)")) -> (element=w250:dbl[])  [unwired: 1 in]
    n154 = call "pumpsec_09_P2.vi"("reset"=w246, "master"=w240, "manual"=w221, "pause"=w248, "Array"=w7, "Target"=w251, "fr_manual"="Grams / min", "Time"=w250) -> ("pumpCtrl"=w129:dbl, "totaltarget"=→"Target":dbl, "target_step"=→"Target amount":dbl, "REGLO D"=w98:dbl, "time_to_target"=→"Time to target" →"Time to target":dbl, "step_fr"=w148:dbl, "amount_step"=→"Amount now" →"Step amount now":dbl, "Scale"=w144:dbl, "elapsed_step"=→"Elapsed / step":dbl, "params"=w241:dbl[])  [unwired: 8 in, 2 out]
    "Scale weight" <- w144
    "Flow rate" <- w148
    "Scale reading" <- w144
    "Flow rate (g/min)" <- w148
    "RPM" <- w98
    n155 = Greater?(x=w129, y=70.0) -> (0:→"PUMP2":bool)
    n156 = Index Array(array=w241, index=1) -> (element=w244:dbl)
    n157 = Index Array(array=w241, index=2) -> (element=→"Amount now" →"Total amount now":dbl)
    n158 = Merge Signals(w144, w148) -> (w155:dynamicdata)
    "Waveform Chart 11" <- w155
    "Waveform Chart 10" <- w155
    n159 = Add(x=1.0, y=w244) -> (x+y=w238:dbl)
    "Current step" <- w238
    n160 = call "STEPINDICATOR_091_2.vi"("current step"=w238, "enable"=i16 1, "manual"=w221) -> ("Led 8"=→"Led8":bool, "Led 10"=→"Led10":bool, "Led 11"=→"Led11":bool, "Led 7"=→"Led7":bool, "Led 1"=→"Led1":bool, "Led 6"=→"Led6":bool, "Led 2"=→"Led2":bool, "Led 12"=→"Led11":bool, "Led 5"=→"Led5":bool, "Led 4"=→"Led4":bool, "Led 3"=→"Led3":bool, "Led 9"=→"Led9":bool)  [unwired: 1 in]
    n161 = Boolean To (0,1)(Boolean="?") -> (0, 1=w215:i16)
    n162 = Boolean To (0,1)(Boolean="?") -> (0, 1=w214:i16)
    n163 = Boolean To (0,1)(Boolean="MASTER CONTROL") -> (0, 1=w216:i16)
    n164 = Boolean To (0,1)(Boolean="Reset 4") -> (0, 1=w196:i16)
    n165 = Index Array(array="PumpSeq 3", index (col)=0 ("disabled index (col)")) -> (element=w199:dbl[])  [unwired: 1 in]
    n166 = Index Array(array="PumpSeq 3", index (col)=1 ("disabled index (col)")) -> (element=w198:dbl[])  [unwired: 1 in]
    n167 = call "pumpsec_09_P3.vi"("reset"=w196, "master"=w216, "manual"=w215, "pause"=w214, "Array"=w7, "Target"=w199, "fr_manual"="Grams / min", "Time"=w198) -> ("pumpCtrl"=w126:dbl, "totaltarget"=→"Target":dbl, "target_step"=→"Target amount":dbl, "REGLO D"=w97:dbl, "time_to_target"=→"Time to target" →"Time to target":dbl, "step_fr"=w147:dbl, "amount_step"=→"Amount now" →"Step amount now":dbl, "Scale"=w143:dbl, "elapsed_step"=→"Elapsed / step":dbl, "params"=w189:dbl[])  [unwired: 8 in, 2 out]
    "Scale weight" <- w143
    "Flow rate" <- w147
    "Scale reading" <- w143
    "Flow rate (g/min)" <- w147
    "RPM" <- w97
    n168 = Greater?(x=w126, y=70.0) -> (0:→"PUMP3":bool)
    n169 = Merge Signals(w145, w144, w143) -> (→"Waveform Chart 7":dynamicdata)
    n170 = Index Array(array=w189, index=1) -> (element=w190:dbl)
    n171 = Index Array(array=w189, index=2) -> (element=→"Amount now" →"Total amount now":dbl)
    n172 = Add(x=1.0, y=w190) -> (x+y=w188:dbl)
    "Current step" <- w188
    n173 = call "Convert to Dynamic Data4"("2D Array"="PumpSeq 3") -> ("Dynamic Data Type"=w102:dynamicdata)  [unwired: 3 in]
    n174 = call "Convert to Dynamic Data3"("2D Array"="PumpSeq 2") -> ("Dynamic Data Type"=w104:dynamicdata)  [unwired: 3 in]
    n175 = call "Convert to Dynamic Data2"("2D Array"="PumpSeq 4") -> ("Dynamic Data Type"=w107:dynamicdata)  [unwired: 3 in]
    n176 = Merge Signals(w102, w104, w107) -> (w106:dynamicdata)
    n177 = Merge Signals(w143, w147) -> (w152:dynamicdata)
    "Waveform Chart 13" <- w152
    "Waveform Chart 12" <- w152
    n178 = Boolean To (0,1)(Boolean="Save Seq") -> (0, 1=w101:i16)
    n179 = for {
      N: w101 -> [_]
      tunnel: w106 -> [w388]
      tunnel: "Configuration file" -> [w389]
      tunnel: "Save Seq" -> [w387]
      n180 = call "Write To Measurement File2"("Signals"=w388, "Reset"=w387, "Filename"=w389) -> ()  [unwired: 14 in, 3 out]
    }
    n181 = call "STEPINDICATOR_091_4.vi"("current step"=w188, "enable"=i16 1, "manual"=w215) -> ("Led 8"=→"Led8 2":bool, "Led 10"=→"Led10 2":bool, "Led 11"=→"Led11 2":bool, "Led 7"=→"Led7 2":bool, "Led 1"=→"Led1 2":bool, "Led 6"=→"Led6 2":bool, "Led 2"=→"Led2 2":bool, "Led 12"=→"Led11 3":bool, "Led 5"=→"Led5 2":bool, "Led 4"=→"Led4 2":bool, "Led 3"=→"Led3 2":bool, "Led 9"=→"Led9 2":bool)  [unwired: 1 in]
    n182 = call "MWriteRS232_1.vi"("P3"=w97, "P2"=w98, "P1"=w99, "LAUDA"=w81) -> ()  [unwired: 8 in]
    n183 = Merge Signals(w153, w155, w152) -> (w151:dynamicdata)
    n184 = Boolean To (0,1)(Boolean="Read Seq") -> (0, 1=w100:i16)
    n185 = for {
      N: w100 -> [_]
      tunnel: "Configuration file" -> [w360]
      tunnel: "Read Seq" -> [w359]
      n186 = while {
        tunnel: [w386] -> w382
        tunnel: w360 -> [w385]
        tunnel: w359 -> [w383]
        stop <- w384 stop-if-true
        n187 = call "Read From Measurement File"("Filename"=w385, "Reset"=w383) -> ("Signals"=w386:dynamicdata, "EOF?"=w384:bool)  [unwired: 4 in, 4 out]
      }
      n188 = call "Convert from Dynamic Data"("Dynamic Data Type"=w382) -> ("Array"=w372:dbl[][])  [unwired: 3 in]
      "Config File" <- w372
      n189 = Array Subset(array=w372, index (row)=20 ("index"), length (row)=10 ("length")) -> (w379:dbl[][])  [unwired: 2 in]
      n190 = Array Subset(array=w372, index (row)=10 ("index"), length (row)=10 ("length")) -> (w374:dbl[][])  [unwired: 2 in]
      n191 = Array Subset(array=w372, index (row)=0 ("index"), length (row)=10 ("length")) -> (w373:dbl[][])  [unwired: 2 in]
      n192 = Array Subset(array=w372, index (row)=30 ("index"), length (row)=8 ("length")) -> (w361:dbl[][])  [unwired: 2 in]
      n193 = property on="PumpSeq 4" class="Arr (strict)"("Val(Sgnl)"=w379) -> ()  [unwired: 2 in, 2 out]
      n194 = property on="PumpSeq 2" class="Arr (strict)"("Val(Sgnl)"=w374) -> ()  [unwired: 2 in, 2 out]
      n195 = property on="PumpSeq 3" class="Arr (strict)"("Val(Sgnl)"=w373) -> ()  [unwired: 2 in, 2 out]
      n196 = Index Array(array=w361, index (row)=2, index (col)=0 ("disabled index (col)")) -> ()  [unwired: 1 out]
      n197 = Index Array(array=w361, index (row)=4, index (col)=0 ("disabled index (col)")) -> ()  [unwired: 1 out]
      n198 = Index Array(array=w361, index (row)=0, index (col)=1 ("disabled index (col)")) -> ()  [unwired: 1 out]
      n199 = Index Array(array=w361, index (row)=1, index (col)=1 ("disabled index (col)")) -> ()  [unwired: 1 out]
    }
    n200 = Merge Signals(w150, w151, w2) -> (w38:dynamicdata)
    n201 = call "Build Table"("Include time data"=TRUE, "Signals"=w38) -> ("Table"=w269:string[][])  [unwired: 3 in, 6 out]
    n202 = Delete From Array(array=w269, length=13, index (col)=0 ("index (row)")) -> (array with subset deleted=→"Table":string[][])  [unwired: 1 in, 1 out]
    n203 = call "filenameparser_09.vi"("Description"="Description", "start path"="Browse folder", "Project name"="Project name", "User (initials)"="User (initials)", "OK Button in"="OK Button 2") -> ("appended path 2"=w82:path, "appended path"=w265:path)  [unwired: 4 in, 1 out]
    "Output File" <- w82
    n204 = Boolean To (0,1)(Boolean="OK Button") -> (0, 1=w264:i16)
    n205 = for {
      N: w264 -> [_]
      tunnel: w265 -> [w351]
      w355 = " " ("string")
      n206 = property on="Add comment" class="Str"("Val(Sgnl)"="" ("Value (Signaling)")) -> ()  [unwired: 2 in, 2 out]
      n207 = Get Date/Time String(want seconds? (F)=TRUE) -> (date string=w358:string, time string=w356:string)  [unwired: 2 in]
      n208 = Concatenate Strings(w358, w355, w356, w355, "Add comment") -> (w354:string)
      n209 = feedback #8() -> (w353:string[])  [unwired: 1 in]
      n210 = Build Array (concatenate)(w353, w354) -> (w352:string[])
      n211 = feedback-in #8(w352) -> ()
      n212 = Write to Text File(file (use dialog)=w351, text=w352) -> ()  [unwired: 2 in, 3 out]
    }
    n213 = call "Header Names 4.vi"("Dynamic Data"=w38) -> ("Signals Out"=w39:dynamicdata)  [unwired: 10 in]
    n214 = call "Write To Measurement File"("Signals"=w39, "Enable"="OK Button 2", "Filename"=w82) -> ()  [unwired: 14 in, 3 out]
    "Boolean" <- "OK Button 2"
  }
